vi "Get Samples and Timeout from Task Timing.vi"(8 "error in":errorcluster, 11 "task in":refnum<k21>) -> (0 "error out":errorcluster, 1 "timeout":dbl, 2 "samples":i32, 3 "task out":refnum<k21>)   [LabVIEW 2024, in "DSA_CFG_ACQ.lvlib"]
uses:
  DSA_CFG_ACQ.lvlib
  <resource>/objmgr/daqmx.rc
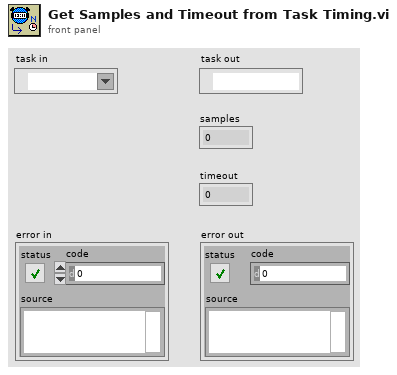
[diagram p1: front panel]
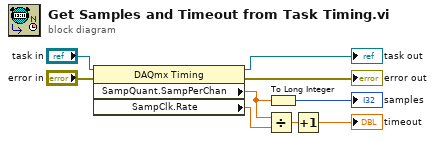
[diagram p0: block diagram]
diagram:
  n1 = property class="DAQmx Timing"(reference="task in", error in="error in") -> (reference out=→"task out":refnum<k21>, error out=→"error out":errorcluster, "SampQuant.SampPerChan"=w4:dbl, "SampClk.Rate"=w5:dbl)
  n2 = Divide(x=w4, y=w5) -> (x/y=w6:dbl)
  n3 = To Long Integer(number=w4) -> (32bit integer=→"samples":i32)
  n4 = Increment(x=w6) -> (x+1=→"timeout":dbl)
